vi "Read MotionData.vi"(8 "error in (no error)":errorcluster, 10 "ReadSize":u32, 11 "AODAcq in":refnum<class "AODAcq.lvclass">) -> (0 "error out":errorcluster, 2 "MotionData":waveform(i32)[](array[waveform]), 3 "AODAcq out":refnum<class "AODAcq.lvclass">)   [LabVIEW 2014, in "AODAcq.lvclass"]
uses:
  AODAcq.lvclass
  AODAcq.lvclass/AODAcq.ctl
  <vilib>/Utility/error.llb/Error Cluster From Error Code.vi
  <vilib>/rvi/errors/niLvFpgaAdjustHostInterfaceError.vi
  HDF5Tools/LabView/Append To Dataset 2D Double.vi
  <vilib>/rvi/interface/nirviMethod/nirviMethod.xnode
  FPGA_Control/AODRef.ctl
  FPGA Bitfiles/AodScanner_FPGATarget_AODControl(FPGA)_TyJc9yYmyGA.lvbitx
  HDF5Tools/LabView/HDF5Tools.lvlib
  <vilib>/rvi/errors/niLvFpgaMergeErrorWithErrorCode.vi
  <vilib>/FPGAPlugInAG/PXIe-7965R/niLvFpga_ReadFifo_PXIe-7965R.vi
panel:
  out "Samples":i32
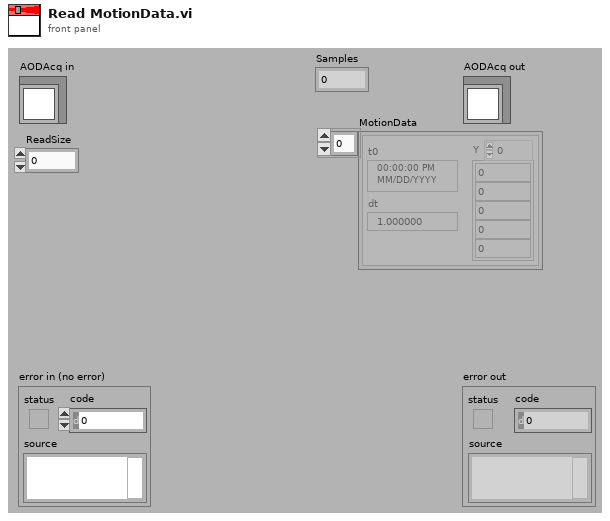
[diagram p1: front panel]
types:
  T1 = typedef "AODRef.ctl" = refnum<k20>
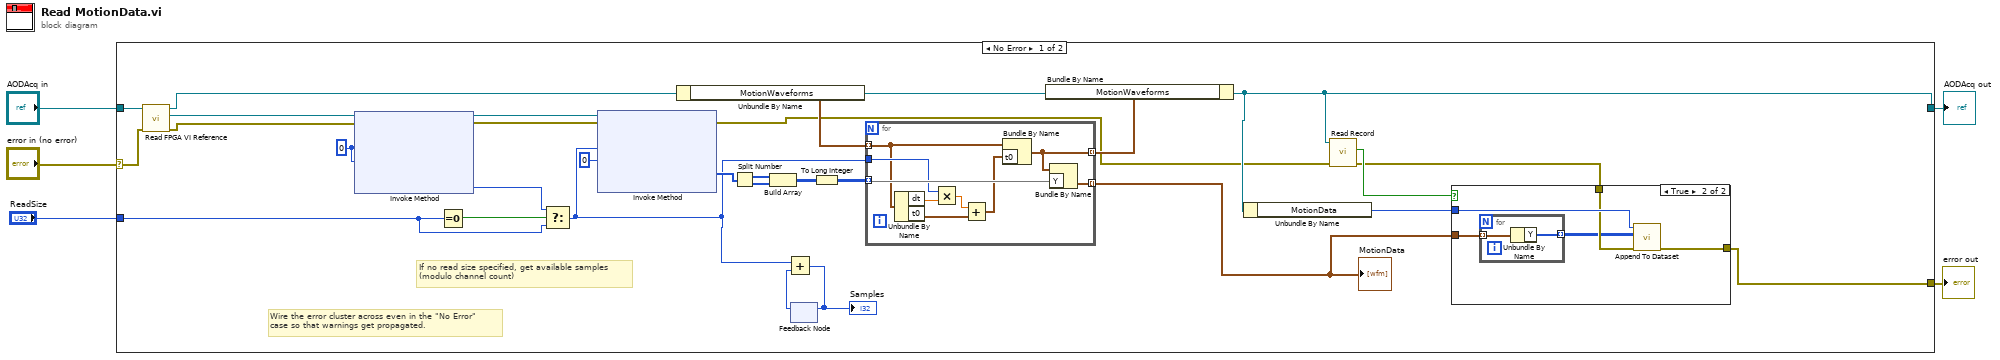
[diagram p0: block diagram]
diagram:
  n1 = case shown="No Error" "error in (no error)" {
    selector: "error in (no error)" -> [w28 w53]
    tunnel: [w9 w53] -> w4
    tunnel: [w10 w52] -> w2
    tunnel: "AODAcq in" -> [w34 w52]
    tunnel: "ReadSize" -> [w14 _]
    frame No Error {
      w33 = u32 0 ("Number of Elements")
      # "If no read size specified, get available samples \n(modulo channel count)"
      # "Wire the error cluster across even in the \"No Error\"\ncase so that warnings get propagated."
      n2 = call-dynamic "Read FPGA VI Reference.vi"("error in (no error)"=w28, "AODAcq in"=w34) -> ("error out"=w15:errorcluster, "FPGA VI Reference"=w16:T1, "AODAcq out"=w26:refnum<class "AODAcq.lvclass">)  [unwired: 7 in]
      n3 = xnode "Invoke Method"("FPGA VI Reference In"=w16, "error in"=w15, "Number of Elements"=w33, "Timeout (ms)"=w33) -> ("FPGA VI Reference Out"=w31:T1, "error out"=w30:errorcluster, "Elements Remaining"=w13:u32)  [unwired: 1 out]
      n4 = Equal To 0?(x=w14) -> (x = 0?=w32:bool)
      n5 = Select(t=w13, s=w32, f=w14) -> (s? t:f=w17:u32)
      n6 = xnode "Invoke Method"("FPGA VI Reference In"=w31, "error in"=w30, "Number of Elements"=w17, "Timeout (ms)"=0) -> ("error out"=w7:errorcluster, "Data"=w19:u64[])  [unwired: 2 out]
      n7 = Unbundle By Name(w26) -> ("MotionWaveforms"=w27:waveform(i32)[])
      n8 = Split Number(x=w19) -> (hi(x)=w21:u32[], lo(x)=w22:u32[])
      n9 = Build Array(w21, w22) -> (w20:u32[][])
      n10 = feedback #1() -> (w23:u32)  [unwired: 1 in]
      n11 = Add(x=w17, y=w23) -> (x+y=w24:u32)
      "Samples" <- w24
      n12 = feedback-in #1(w24) -> ()
      n13 = To Long Integer(number=w20) -> (32bit integer=w18:i32[][])
      n14 = for {
        tunnel: w18 -> [w51] mode=indexing
        tunnel: [w50] -> w8 mode=indexing
        tunnel: w27 -> [w45] mode=indexing
        tunnel: w17 -> [w48]
        tunnel: [w43] -> w25 mode=indexing
        n15 = Unbundle By Name(w45) -> ("dt"=w49:dbl, "t0"=w46:timestamp)
        n16 = Multiply(x=w48, y=w49) -> (x*y=w47:dbl)
        n17 = Add(x=w47, y=w46) -> (x+y=w44:timestamp)
        n18 = Bundle By Name(cluster=w45, "t0"=w44) -> (w43:waveform(i32))
        n19 = Bundle By Name(cluster=w43, "Y"=w51) -> (w50:waveform(i32))
      }
      "MotionData" <- w8
      n20 = Bundle By Name(cluster=w26, "MotionWaveforms"=w25) -> (w10:refnum<class "AODAcq.lvclass">)
      n21 = Unbundle By Name(w10) -> ("MotionData"=w12:i32)
      n22 = call-dynamic "Read Record.vi"("error in (no error)"=w7, "AODAcq in"=w10) -> ("error out"=w6:errorcluster, "Record"=w11:bool)  [unwired: 7 in, 1 out]
      n23 = case shown="True" w11 {
        tunnel: w12 -> [_ w40]
        tunnel: [w35 w39] -> w9
        tunnel: w8 -> [_ w38]
        tunnel: w6 -> [w35 w37]
        frame False {
        }
        frame True {
          n24 = for {
            tunnel: [w42] -> w36 mode=indexing
            tunnel: w38 -> [w41] mode=indexing
            n25 = Unbundle By Name(w41) -> ("Y"=w42:i32[])
          }
          n26 = call-poly "Append To Dataset.vi"("Error in (no error)"=w37, "Data"=w36, "Dataset id in"=w40) -> ("Error out"=w39:errorcluster)  [unwired: 7 in, 1 out]
        }
      }
    }
    frame Error {
    }
  }
  "error out" <- w4
  "AODAcq out" <- w2
